vi "readI.vi"(2 "SMU":dbl, 3 "*VISA resource name*":refnum<visa-resource-name>="GPIB0::16::INSTR") -> (0 "current":dbl format="%#_13g", 1 "*VISA resource name*DUP":refnum<visa-resource-name>="GPIB0::17::INSTR")   [LabVIEW 2023]
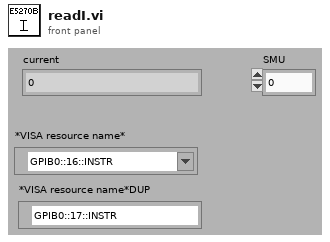
[diagram p1: front panel]
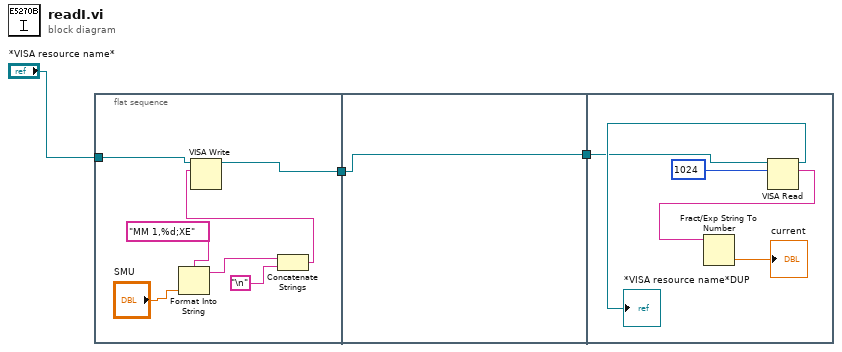
[diagram p0: block diagram]
diagram:
  n1 = flat-sequence {
    tunnel: "*VISA resource name*" -> [w10]
    tunnel: [w7] -> w2
    tunnel: w2 -> [w11]
    tunnel: [w11] -> w1
    tunnel: w1 -> [w12]
    frame #0 {
      n2 = Format Into String(format string="MM 1,%d;XE", "SMU") -> (resulting string=w4:string)  [unwired: 2 in, 1 out]
      n3 = Concatenate Strings(w4, "\n") -> (w8:string)
      n4 = VISA Write(VISA resource name=w10, write buffer=w8) -> (VISA resource name out=w7:refnum<visa-resource-name>)  [unwired: 1 in, 2 out]
    }
    frame #1 {
    }
    frame #2 {
      n5 = VISA Read(VISA resource name=w12, byte count=1024) -> (VISA resource name out=→"*VISA resource name*DUP":refnum<visa-resource-name>, read buffer=w15:string)  [unwired: 1 in, 2 out]
      n6 = Fract/Exp String To Number(string=w15) -> (number=→"current":dbl)  [unwired: 4 out]
    }
  }
